vi "Role_Auto_Secim.vi"(8 "Activate":bool, 11 "Denge Kolu":u16(ring) items=["Default", "Ana Denge", "Wagner", "10R", "1R"]) -> ()   [LabVIEW 2014]
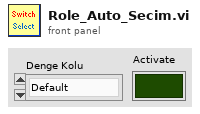
[diagram p1: front panel]
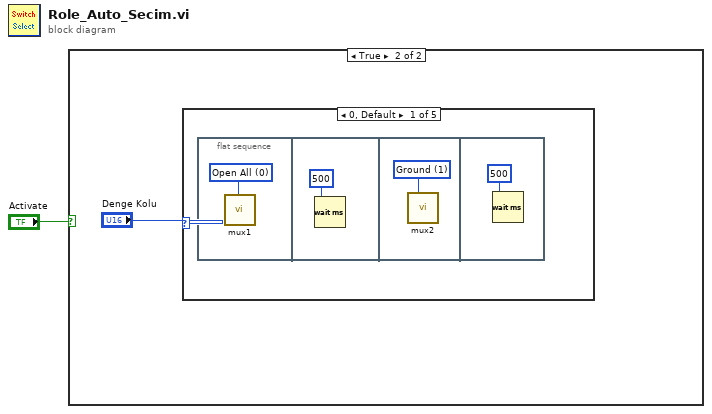
[diagram p0: block diagram]
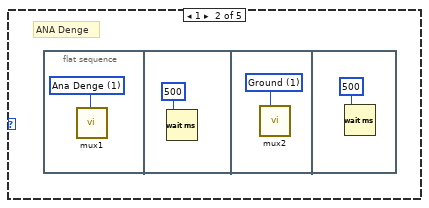
[diagram p3: hidden frame]
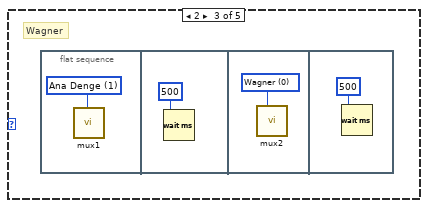
[diagram p4: hidden frame]
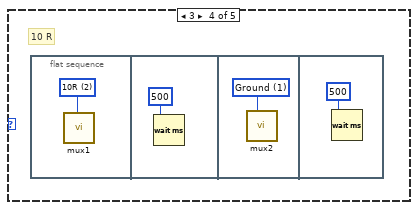
[diagram p5: hidden frame]
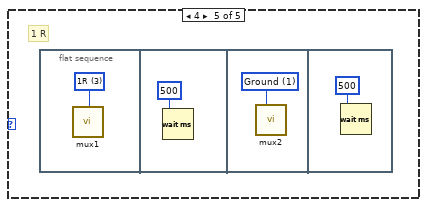
[diagram p6: hidden frame]
diagram:
  n1 = case shown="True" "Activate" {
    frame False {
    }
    frame True {
      n2 = case shown="0, Default" "Denge Kolu" {
        frame 0, Default {
          n3 = flat-sequence {
            frame #0 {
              w3 = u16 0 items=["Open All", "Ana Denge", "10R", "1R"] ("Ring")
              n4 = call "mux1.vi"("Ring"=w3) -> ()  [unwired: 9 in, 1 out]
            }
            frame #1 {
              n5 = Wait (ms)(milliseconds to wait=u32 500) -> ()  [unwired: 1 out]
            }
            frame #2 {
              w5 = u16 1 items=["Wagner", "Ground"] ("Switch")
              n6 = call "mux2.vi"("Switch"=w5) -> ()  [unwired: 7 in, 1 out]
            }
            frame #3 {
              n7 = Wait (ms)(milliseconds to wait=u32 500) -> ()  [unwired: 1 out]
            }
          }
        }
        frame 1 {
          # "ANA Denge"
          n8 = flat-sequence {
            frame #0 {
              w7 = u16 1 items=["Open All", "Ana Denge", "10R", "1R"] ("Ring")
              n9 = call "mux1.vi"("Ring"=w7) -> ()  [unwired: 9 in, 1 out]
            }
            frame #1 {
              n10 = Wait (ms)(milliseconds to wait=u32 500) -> ()  [unwired: 1 out]
            }
            frame #2 {
              w9 = u16 1 items=["Wagner", "Ground"] ("Switch")
              n11 = call "mux2.vi"("Switch"=w9) -> ()  [unwired: 7 in, 1 out]
            }
            frame #3 {
              n12 = Wait (ms)(milliseconds to wait=u32 500) -> ()  [unwired: 1 out]
            }
          }
        }
        frame 2 {
          # "Wagner"
          n13 = flat-sequence {
            frame #0 {
              w11 = u16 1 items=["Open All", "Ana Denge", "10R", "1R"] ("Ring")
              n14 = call "mux1.vi"("Ring"=w11) -> ()  [unwired: 9 in, 1 out]
            }
            frame #1 {
              n15 = Wait (ms)(milliseconds to wait=u32 500) -> ()  [unwired: 1 out]
            }
            frame #2 {
              w13 = u16 0 items=["Wagner", "Ground"] ("Switch")
              n16 = call "mux2.vi"("Switch"=w13) -> ()  [unwired: 7 in, 1 out]
            }
            frame #3 {
              n17 = Wait (ms)(milliseconds to wait=u32 500) -> ()  [unwired: 1 out]
            }
          }
        }
        frame 3 {
          # "10 R"
          n18 = flat-sequence {
            frame #0 {
              w15 = u16 2 items=["Open All", "Ana Denge", "10R", "1R"] ("Ring")
              n19 = call "mux1.vi"("Ring"=w15) -> ()  [unwired: 9 in, 1 out]
            }
            frame #1 {
              n20 = Wait (ms)(milliseconds to wait=u32 500) -> ()  [unwired: 1 out]
            }
            frame #2 {
              w17 = u16 1 items=["Wagner", "Ground"] ("Switch")
              n21 = call "mux2.vi"("Switch"=w17) -> ()  [unwired: 7 in, 1 out]
            }
            frame #3 {
              n22 = Wait (ms)(milliseconds to wait=u32 500) -> ()  [unwired: 1 out]
            }
          }
        }
        frame 4 {
          # "1 R"
          n23 = flat-sequence {
            frame #0 {
              w19 = u16 3 items=["Open All", "Ana Denge", "10R", "1R"] ("Ring")
              n24 = call "mux1.vi"("Ring"=w19) -> ()  [unwired: 9 in, 1 out]
            }
            frame #1 {
              n25 = Wait (ms)(milliseconds to wait=u32 500) -> ()  [unwired: 1 out]
            }
            frame #2 {
              w21 = u16 1 items=["Wagner", "Ground"] ("Switch")
              n26 = call "mux2.vi"("Switch"=w21) -> ()  [unwired: 7 in, 1 out]
            }
            frame #3 {
              n27 = Wait (ms)(milliseconds to wait=u32 500) -> ()  [unwired: 1 out]
            }
          }
        }
      }
    }
  }
